vi "Scratch.vi"() -> ()   [LabVIEW 2020, in "VolatusSeq.lvlib"]
uses:
  VolatusSeq.lvlib
  Sequencing Status JSON.ctl
  Sequence Status JSON.ctl
  lv-web-crypto/lv-crypto/Crypto/Hashes/SHA-256/SHA-256.lvclass
  <vilib>/httpClient/MultipartData.ctl
  839e7588-aafe-4656-a2fc-0ebd197a9b7a.vi
  9333b484-011f-4693-912f-1257e8b2ee91.vi
  d0b18555-7aa2-4285-8466-e3de5a6bf30b.vi
  80ab21ca-ea82-40af-a504-7941cea15b69.vi
  <vilib>/JDP Science/JSONtext/Next JSON Value.vi
  <vilib>/JDP Science/JSONtext/String Subset.vi
  <vilib>/JDP Science/JSONtext/Parsing/Advance past next JSON Value (inlined COPY).vi
  <vilib>/JDP Science/JSONtext/Parsing/Advance past whitespace.vi
  <vilib>/JDP Science/JSONtext/Parsing/Advance past String.vi
  <vilib>/JDP Science/JSONtext/Parsing/Advance past Number.vi
  <vilib>/JDP Science/JSONtext/Parsing/Advance past Line Ending.vi
  <vilib>/JDP Science/JSONtext/Parsing/Parse Full Path or Item Name.vi
  <vilib>/JDP Science/JSONtext/Parsing/Advance past Array.vi
  <vilib>/JDP Science/JSONtext/Parsing/Advance past Object.vi
  <vilib>/JDP Science/JSONtext/support/Error Cluster From Code.vi
  <vilib>/JDP Science/JSONtext/Offset/Find Item Locations by Path.vi
  <vilib>/JDP Science/JSONtext/JSON text to Variant.vi
  <vilib>/JDP Science/JSONtext/LVClass Serializer/JSONtext LVClass Serializer.lvclass
  <vilib>/JDP Science/JSONtext/JSONtext.lvlib
  lv-web-crypto/lv-crypto/Crypto/Crypto.lvlib
  <vilib>/httpClient/LabVIEWHTTPClient.lvlib
  lv-vecto/Vecto/Vecto.lvlib
  lv-web-crypto/lv-json/JSON/JSON.lvlib
  ad4a9e69-8c40-4036-95cd-164e8a1331be.vi
panel:
  in  "URL Base":string
  out "Table":string[][](table)
  in  "Abort":bool
  in  "Unload":bool
  in  "Start":bool
  in  "Load":bool
  in  "VSEQ":string="{\n    \"Sequence\": {\n        \"Name\": \"Bottle Condition\",\n        \"Version\": \"1\",\n        \"Comment\": \"Control state machine for bottle heating/cooling.\",\n        \"Entry\": \"Start\",\n        \"Abort\": \"Stop\",\n        \"States\": {\n            \"Start\": {\n                \"Comment\": \"Reset bottle controls to off state.\",\n                \"Steps\": [\n                    {\n                        \"Time\": 0,\n                        \"Commands\": [\n                            {\"Type\": \"Transition\", \"Target\": \"Hold\"}\n                        ]\n                    }\n                ]\n            },\n            \"Hold\": {\n                \"Comment\": \"Bottle in range, controls off.\",\n                \"Steps\": [\n                    {\n                        \"Time\": 0,\n                        \"Commands\": [\n                            {\"Type\": \"Digital\", \"Channel\": \"BottleCool\", \"Value\": false},\n                            {\"Type\": \"Digital\", \"Channel\": \"BottleHeat\", \"Value\": false}\n                        ]\n                    }\n                ],\n                \"Transitions\": [\n                    {\n                        \"Type\": \"State\",\n                        \"Target\": \"Cool\",\n                        \"Logic\": \"Any\",\n                        \"Conditions\": [\n                            {\"Type\": \"HighLimit\", \"Channel\": \"BottlePSI\", \"Limit\": 850}\n                        ]\n                    },\n                    {\n                        \"Type\": \"State\",\n                        \"Target\": \"Heat\",\n                        \"Logic\": \"Any\",\n                        \"Conditions\": [\n                            {\"Type\": \"LowLimit\", \"Channel\": \"BottlePSI\", \"Limit\": 750}\n                        ]\n                    }\n                ]\n            },\n            \"Cool\": {\n                \"Comment\": \"Cooling, wait for pressure to drop.\",\n                \"Steps\": [\n                    {\n                        \"Time\": 0,\n                        \"Commands\": [\n                            {\"Type\": \"Digital\", \"Channel\": \"BottleCool\", \"Value\": true}\n                        ]\n                    }\n                ],\n                \"Transitions\": [\n                    {\n                        \"Type\": \"State\",\n                        \"Target\": \"Start\",\n                        \"Logic\": \"Any\",\n                        \"Conditions\": [\n                            {\"Type\": \"LowLimit\", \"Channel\": \"BottlePSI\", \"Limit\": 800}\n                        ]\n                    }\n                ]\n            },\n            \"Heat\": {\n                \"Comment\": \"Heating, wait for pressure to rise.\",\n                \"Steps\": [\n                    {\n                        \"Time\": 0,\n                        \"Commands\": [\n                            {\"Type\": \"Digital\", \"Channel\": \"BottleHeat\", \"Value\": true}\n                        ]\n                    }\n                ],\n                \"Transitions\": [\n                    {\n                        \"Type\": \"State\",\n                        \"Target\": \"Start\",\n                        \"Logic\": \"Any\",\n                        \"Conditions\": [\n                            {\"Type\": \"HighLimit\", \"Channel\": \"BottlePSI\", \"Limit\": 800}\n                        ]\n                    }\n                ]\n            },\n            \"Stop\": {\n                \"Comment\": \"Stopping, ensure controls off.\",\n                \"Steps\": [\n                    {\n                        \"Time\": 0,\n                        \"Commands\": [\n                            {\"Type\": \"Digital\", \"Channel\": \"BottleCool\", \"Value\": false},\n                            {\"Type\": \"Digital\", \"Channel\": \"BottleHeat\", \"Value\": false}\n                        ]\n                    }\n                ]\n            }\n        }\n    }\n}"
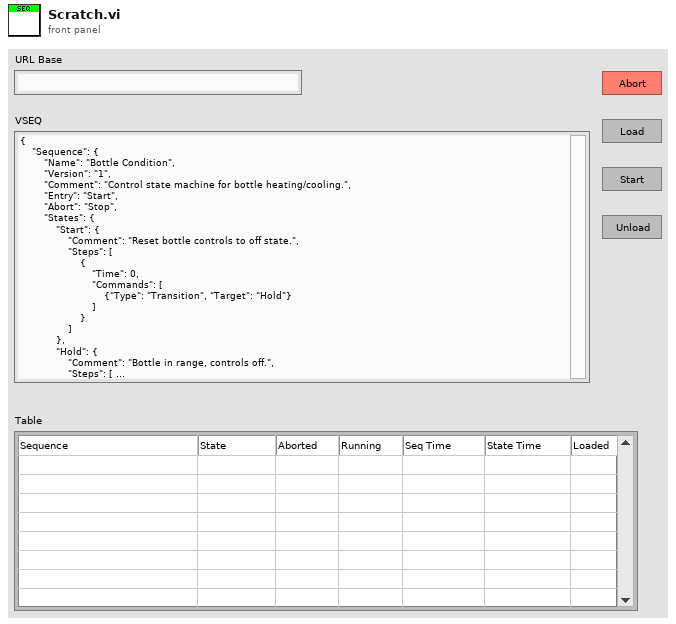
[diagram p1: front panel]
types:
  T1 = typedef "VolatusSeq.lvlib/Sequencing Status JSON.ctl" = cluster{"sequences":T2[]}
  T2 = typedef "VolatusSeq.lvlib/Sequence Status JSON.ctl" = cluster{"name":string, "state":string, "running":bool, "abort":bool, "time":cluster{"seq":i64, "state":i64, "wall":i64}, "loaded":bool}
  T3 = typedef "LabVIEWHTTPClient.lvlib/MultipartData.ctl" = cluster{"Name":string, "Value":string, "File":path, "Filename":string, "MIME type":string}
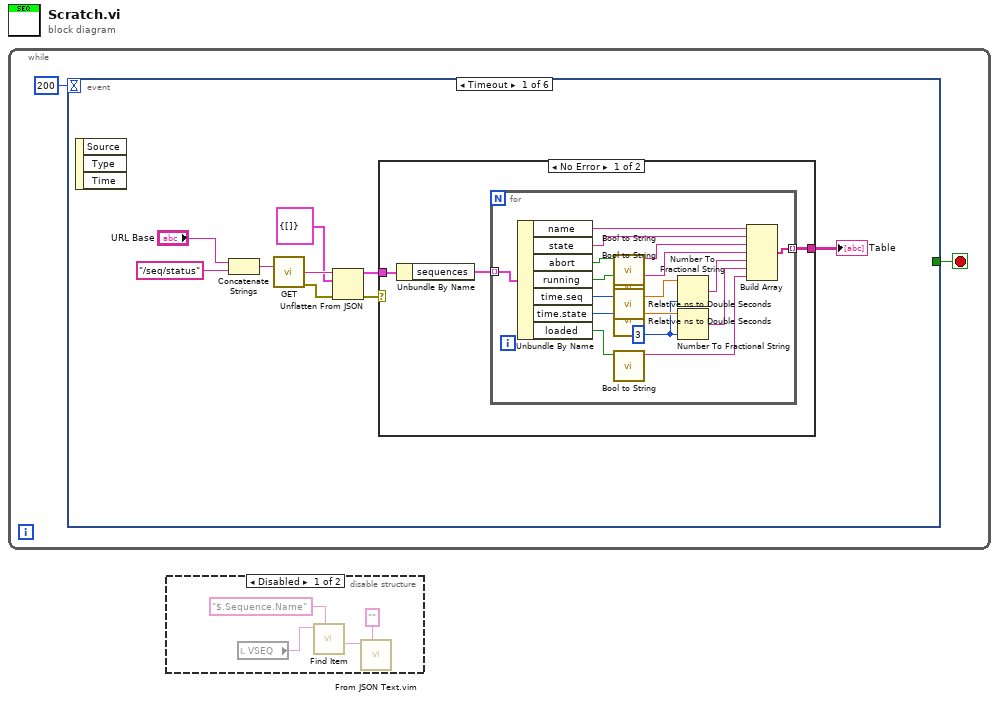
[diagram p0: block diagram]
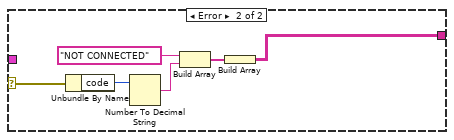
[diagram p3: hidden frame]
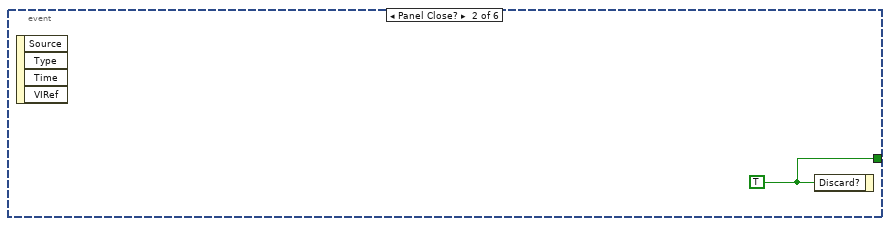
[diagram p4: hidden frame]
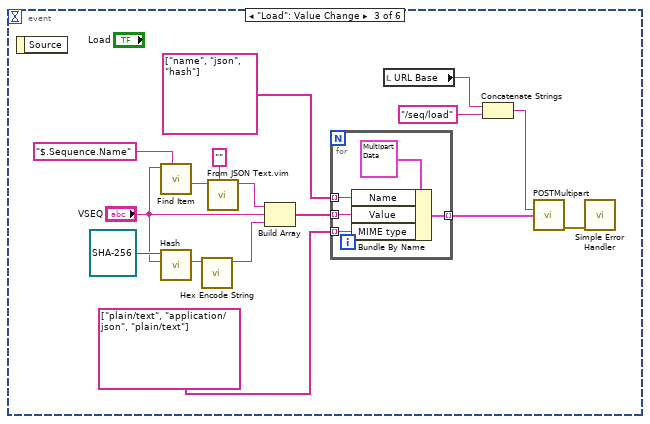
[diagram p5: hidden frame]
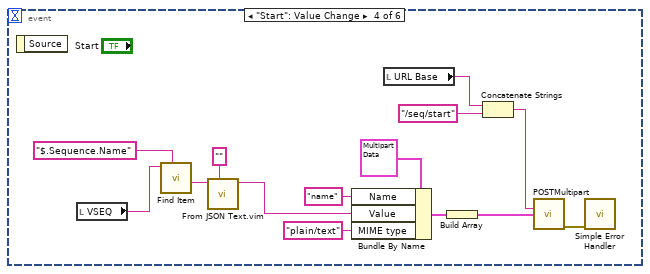
[diagram p6: hidden frame]
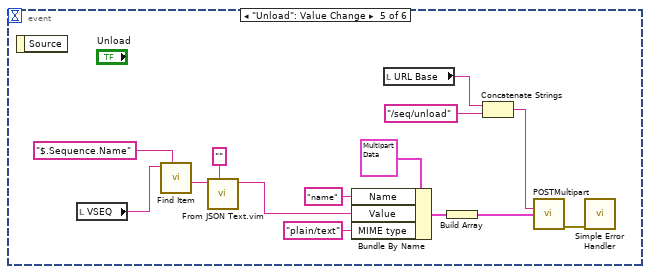
[diagram p7: hidden frame]
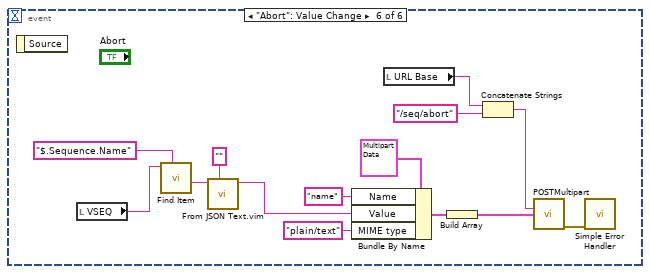
[diagram p8: hidden frame]
diagram:
  n1 = while {
    stop <- w1 stop-if-true
    n2 = event shown="[0] Timeout" {
      selector: _ -> [_ _ _ _ _ _]
      dyn-events: _ -> [_ _ _ _ _ _]
      timeout: 200 -> [_ _ _ _ _ _]
      tunnel: [_ w38 _ _ _ _] -> w1
      event Timeout {
        n3 = event-data() -> ()  [unwired: 1 in, 3 out]
        n4 = Concatenate Strings("URL Base", "/seq/status" ("string")) -> (w9:string)
        n5 = call <vilib>:"GET.vi"("url"=w9) -> ("body"=w8:string, "error out"=w7:errorcluster)  [unwired: 11 in, 2 out]
        n6 = Unflatten From JSON(JSON string=w8, type and defaults=T1 {"sequences"=[]} ("Sequencing Status JSON"), error in (no error)=w7) -> (value=w5:T1, error out=w3:errorcluster)  [unwired: 4 in]
        n7 = case shown="No Error" w3 {
          selector: w3 -> [_ w37]
          tunnel: w5 -> [w14 _]
          tunnel: [w12 w32] -> w4
          frame No Error {
            n8 = Unbundle By Name(w14) -> ("sequences"=w13:T2[])
            n9 = for {
              tunnel: w13 -> [w31] mode=indexing
              tunnel: [w17] -> w12 mode=indexing
              w25 = i16 3 ("precision (6)")
              n10 = Unbundle By Name(w31) -> ("name"=w23:string, "state"=w22:string, "abort"=w28:bool, "running"=w27:bool, "time.seq"=w30:i64, "time.state"=w29:i64, "loaded"=w16:bool)
              n11 = call "Bool to String.vi"("Boolean"=w28) -> ("Value"=w21:string)  [unwired: 10 in]
              n12 = call "Bool to String.vi"("Boolean"=w27) -> ("Value"=w20:string)  [unwired: 10 in]
              n13 = call "Relative ns to Double Seconds.vi"("relative ns"=w30) -> ("Double s"=w24:dbl)  [unwired: 6 in]
              n14 = call "Relative ns to Double Seconds.vi"("relative ns"=w29) -> ("Double s"=w26:dbl)  [unwired: 6 in]
              n15 = call "Bool to String.vi"("Boolean"=w16) -> ("Value"=w15:string)  [unwired: 10 in]
              n16 = Number To Fractional String(number=w24, precision (6)=w25) -> (F-format string=w19:string)  [unwired: 2 in]
              n17 = Number To Fractional String(number=w26, precision (6)=w25) -> (F-format string=w18:string)  [unwired: 2 in]
              n18 = Build Array(w23, w22, w21, w20, w19, w18, w15) -> (w17:string[])
            }
          }
          frame Error {
            n19 = Unbundle By Name(w37) -> ("code"=w36:i32)
            n20 = Number To Decimal String(number=w36) -> (decimal integer string=w34:string)  [unwired: 1 in]
            n21 = Build Array("NOT CONNECTED", w34) -> (w33:string[])
            n22 = Build Array(w33) -> (w32:string[][])
          }
        }
        "Table" <- w4
      }
      event Panel Close? {
        w38 = TRUE ("Discard?")
        n23 = event-data() -> ()  [unwired: 1 in, 4 out]
        n24 = event-data("Discard?"=w38) -> ()  [unwired: 1 in, 1 out]
      }
      event "Load": Value Change {
        n25 = event-data() -> ()  [unwired: 1 in, 1 out]
        n26 = call <vilib>:"Find Item.vi"("$Path or Item Name"="$.Sequence.Name", "JSON"="VSEQ") -> ("<JSON>"=w54:string)  [unwired: 6 in, 3 out]
        n27 = call-dynamic "Hash.vi"("Message"="VSEQ", "SHA-256 in"=refnum<class "SHA-256.lvclass"> refnum) -> ("Hash"=w53:string)  [unwired: 7 in, 2 out]
        n28 = call "Hex Encode String.vi"("String"=w53) -> ("Hex Encoded String"=w47:string)  [unwired: 10 in]
        n29 = call "From JSON Text.vim"("Data Type and Default Value"="", "JSON"=w54) -> ("Data out"=w49:string)  [unwired: 8 in, 1 out]
        n30 = Build Array(w49, "VSEQ", w47) -> (w46:string[])
        n31 = for {
          tunnel: w46 -> [w58] mode=indexing
          tunnel: string[] ["name", "json", "hash"] -> [w57] mode=indexing
          tunnel: string[] ["plain/text", "application/json", "plain/text"] -> [w56] mode=indexing
          tunnel: [w55] -> w43 mode=indexing
          n32 = Bundle By Name(cluster=T3 {"Name"="", "Value"="", "File"=path "", "Filename"="", "MIME type"="application/octet-stream"} ("Element"), "Name"=w57, "Value"=w58, "MIME type"=w56) -> (w55:T3)
        }
        n33 = local read "URL Base"() -> (w42:string)
        n34 = Concatenate Strings(w42, "/seq/load" ("string")) -> (w40:string)
        n35 = call <vilib>:"POSTMultipart.vi"("url"=w40, "data"=w43) -> ("error out"=w39:errorcluster)  [unwired: 10 in, 3 out]
        n36 = call <vilib>:"Simple Error Handler.vi"("error in (no error)"=w39) -> ()  [unwired: 4 in, 5 out]
      }
      event "Start": Value Change {
        n37 = event-data() -> ()  [unwired: 1 in, 1 out]
        n38 = local read "VSEQ"() -> (w66:string)
        n39 = call <vilib>:"Find Item.vi"("$Path or Item Name"="$.Sequence.Name", "JSON"=w66) -> ("<JSON>"=w73:string)  [unwired: 6 in, 3 out]
        n40 = call "From JSON Text.vim"("Data Type and Default Value"="", "JSON"=w73) -> ("Data out"=w62:string)  [unwired: 8 in, 1 out]
        n41 = Bundle By Name(cluster=T3 {"Name"="", "Value"="", "File"=path "", "Filename"="", "MIME type"="application/octet-stream"} ("Element"), "Name"="name", "Value"=w62, "MIME type"="plain/text") -> (w61:T3)
        n42 = local read "URL Base"() -> (w70:string)
        n43 = Build Array(w61) -> (w60:T3[])
        n44 = Concatenate Strings(w70, "/seq/start" ("string")) -> (w68:string)
        n45 = call <vilib>:"POSTMultipart.vi"("url"=w68, "data"=w60) -> ("error out"=w67:errorcluster)  [unwired: 10 in, 3 out]
        n46 = call <vilib>:"Simple Error Handler.vi"("error in (no error)"=w67) -> ()  [unwired: 4 in, 5 out]
      }
      event "Unload": Value Change {
        n47 = event-data() -> ()  [unwired: 1 in, 1 out]
        n48 = local read "VSEQ"() -> (w80:string)
        n49 = call <vilib>:"Find Item.vi"("$Path or Item Name"="$.Sequence.Name", "JSON"=w80) -> ("<JSON>"=w87:string)  [unwired: 6 in, 3 out]
        n50 = call "From JSON Text.vim"("Data Type and Default Value"="", "JSON"=w87) -> ("Data out"=w76:string)  [unwired: 8 in, 1 out]
        n51 = Bundle By Name(cluster=T3 {"Name"="", "Value"="", "File"=path "", "Filename"="", "MIME type"="application/octet-stream"} ("Element"), "Name"="name", "Value"=w76, "MIME type"="plain/text") -> (w75:T3)
        n52 = local read "URL Base"() -> (w84:string)
        n53 = Build Array(w75) -> (w74:T3[])
        n54 = Concatenate Strings(w84, "/seq/unload" ("string")) -> (w82:string)
        n55 = call <vilib>:"POSTMultipart.vi"("url"=w82, "data"=w74) -> ("error out"=w81:errorcluster)  [unwired: 10 in, 3 out]
        n56 = call <vilib>:"Simple Error Handler.vi"("error in (no error)"=w81) -> ()  [unwired: 4 in, 5 out]
      }
      event "Abort": Value Change {
        n57 = event-data() -> ()  [unwired: 1 in, 1 out]
        n58 = local read "VSEQ"() -> (w94:string)
        n59 = call <vilib>:"Find Item.vi"("$Path or Item Name"="$.Sequence.Name", "JSON"=w94) -> ("<JSON>"=w101:string)  [unwired: 6 in, 3 out]
        n60 = call "From JSON Text.vim"("Data Type and Default Value"="", "JSON"=w101) -> ("Data out"=w90:string)  [unwired: 8 in, 1 out]
        n61 = Bundle By Name(cluster=T3 {"Name"="", "Value"="", "File"=path "", "Filename"="", "MIME type"="application/octet-stream"} ("Element"), "Name"="name", "Value"=w90, "MIME type"="plain/text") -> (w89:T3)
        n62 = local read "URL Base"() -> (w98:string)
        n63 = Build Array(w89) -> (w88:T3[])
        n64 = Concatenate Strings(w98, "/seq/abort" ("string")) -> (w96:string)
        n65 = call <vilib>:"POSTMultipart.vi"("url"=w96, "data"=w88) -> ("error out"=w95:errorcluster)  [unwired: 10 in, 3 out]
        n66 = call <vilib>:"Simple Error Handler.vi"("error in (no error)"=w95) -> ()  [unwired: 4 in, 5 out]
      }
    }
  }
  n67 = disable-structure shown="Disabled" {
    frame Disabled {
      n68 = local read "VSEQ"() -> (w102:string)
      n69 = call <vilib>:"Find Item.vi"("$Path or Item Name"="$.Sequence.Name", "JSON"=w102) -> ("<JSON>"=w103:string)  [unwired: 6 in, 3 out]
      n70 = call "From JSON Text.vim"("Data Type and Default Value"="", "JSON"=w103) -> ()  [unwired: 8 in, 2 out]
    }
    frame Enabled {
    }
  }
